vi "AddConnectionHandler.vi"(8 "error in (no error)":errorcluster, 11 "TCP_Server in":refnum<class "TCP_Server.lvclass">) -> (0 "error out":errorcluster, 3 "TCP_Server out":refnum<class "TCP_Server.lvclass">)   [LabVIEW 2023, in "TCP_Server.lvlib" / "TCP_Server.lvclass"]
uses:
  TCP_Server.lvclass
  TCP_Server_Connection_Handler/TCP_Server_Connection_Handler/TCP_Server_Connection_Handler.lvclass
  TCP_Server.lvclass/TCP_Server.ctl
  TCP_Server_Connection_Handler/TCP_Server_Connection_Handler Messages/Write Connection Information Msg/Write Connection Information Msg.lvclass/Write Connection Information Msg.ctl
  <vilib>/ActorFramework/Message Enqueuer/Message Enqueuer.lvclass/Message Enqueuer.ctl
  <vilib>/ActorFramework/Actor/Actor.lvclass/Actor.ctl
  TCP_Server_Connection_Handler/TCP_Server_Connection_Handler Messages/Write Error Logger's Enqueuer Msg/Write Error Logger's Enqueuer Msg.lvclass/Write Error Logger's Enqueuer Msg.ctl
  <vilib>/ActorFramework/Message Enqueuer/Enqueue.vi
  <vilib>/ActorFramework/Message Enqueuer/Init from Existing Queue.vi
  TCP_Server_Connection_Handler/TCP_Server_Connection_Handler Messages/Write Connection Information Msg/Write Connection Information Msg.lvclass
  TCP_Server_Connection_Handler/TCP_Server_Connection_Handler Messages/Write Error Logger's Enqueuer Msg/Write Error Logger's Enqueuer Msg.lvclass
  TCP_Server_Connection_Handler/TCP_Server_Connection_Handler Messages/FindMessageStart Msg/FindMessageStart Msg.lvclass
  TCP_Server Messages/AddConnectionWindow Msg/AddConnectionWindow Msg.lvclass
  <vilib>/ActorFramework/Message Priority Queue/Priority Enqueue.vi
  <vilib>/ActorFramework/Message Enqueuer/Message Enqueuer.lvclass
  <vilib>/ActorFramework/Actor/Actor.lvclass
  TCP_Server_Connection_Handler/TCP_Server_Connection_Handler Messages/SendWelcome Msg/SendWelcome Msg.lvclass
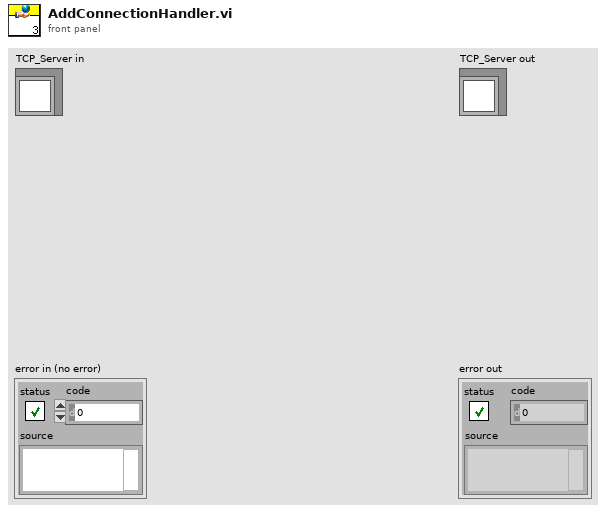
[diagram p1: front panel]
types:
  T1 = typedef "TCP_Server.lvlib/ServerConnection.ctl" = cluster{"Connection Handlers's Enqueuer":refnum<class "Message Enqueuer.lvclass">, "Connection Window's Enqueuer":refnum<class "Message Enqueuer.lvclass">, "Connection Information":T2}
  T2 = typedef "TCP_Listener.lvlib/ConnectionInformation.ctl" = cluster{"Connection number":i32, "Remote Address":string, "Remote Port":u16, "Connection ID":refnum<k5>}
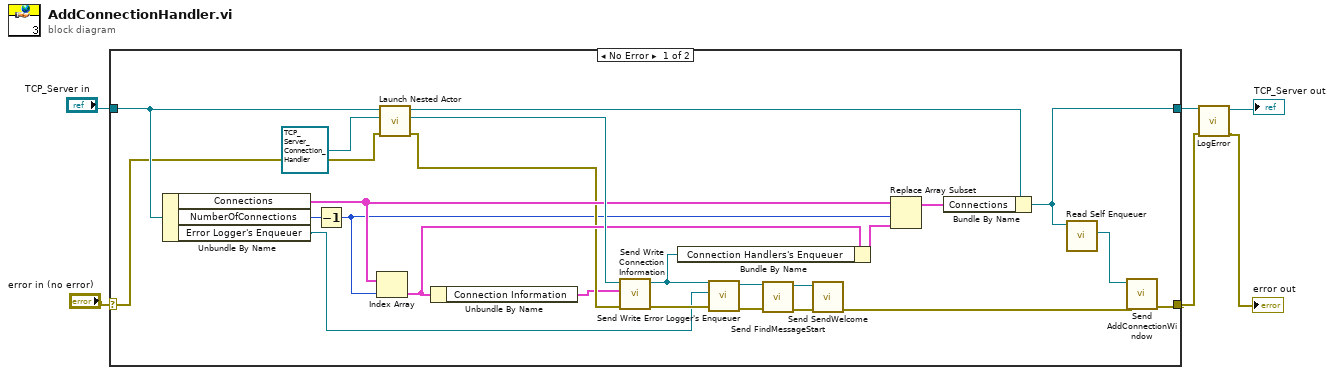
[diagram p0: block diagram]
diagram:
  n1 = case shown="No Error" "error in (no error)" {
    selector: "error in (no error)" -> [w18 w32]
    tunnel: [w20 w32] -> w2
    tunnel: [w19 w31] -> w4
    tunnel: "TCP_Server in" -> [w25 w31]
    frame No Error {
      n2 = Unbundle By Name(w25) -> ("Connections"=w23:T1[], "NumberOfConnections"=w29:i32, "Error Logger's Enqueuer"=w12:refnum<class "Message Enqueuer.lvclass">)
      n3 = Decrement(x=w29) -> (x-1=w15:i32)
      n4 = Index Array(array=w23, index=w15) -> (element=w21:T1)
      n5 = call <vilib>:"Launch Nested Actor.vi"("error in (no error)"=w18, "Nested Actor"=refnum<class "TCP_Server_Connection_Handler.lvclass"> refnum ("TCP_Server_Connection_Handler.lvlib:TCP_Server_Connection_Handler.lvclass"), "Caller Actor in"=w25) -> ("error out"=w17:errorcluster, "Nested Actor's Enqueuer"=w28:refnum<class "Message Enqueuer.lvclass">, "Caller Actor out"=w27:refnum<class "TCP_Server.lvclass">)  [unwired: 6 in]
      n6 = Unbundle By Name(w21) -> ("Connection Information"=w16:T2)
      n7 = call "Send Write Connection Information.vi"("error in (no error)"=w17, "Connection Information"=w16, "Message Enqueuer"=w28) -> ("error out"=w13:errorcluster, "Message Enqueuer out"=w14:refnum<class "Message Enqueuer.lvclass">)  [unwired: 7 in]
      n8 = Bundle By Name(cluster=w21, "Connection Handlers's Enqueuer"=w14) -> (w22:T1)
      n9 = call "Send Write Error Logger's Enqueuer.vi"("error in (no error)"=w13, "Actor Framework:Message Enqueuer"=w12, "Message Enqueuer"=w14) -> ("error out"=w11:errorcluster, "Message Enqueuer out"=w10:refnum<class "Message Enqueuer.lvclass">)  [unwired: 7 in]
      n10 = call "Send FindMessageStart.vi"("error in (no error)"=w11, "Message Enqueuer"=w10) -> ("error out"=w9:errorcluster, "Message Enqueuer out"=w8:refnum<class "Message Enqueuer.lvclass">)  [unwired: 8 in]
      n11 = call "Send SendWelcome.vi"("error in (no error)"=w9, "Message Enqueuer"=w8) -> ("error out"=w7:errorcluster)  [unwired: 8 in, 1 out]
      n12 = Replace Array Subset(array=w23, new element=w22, index=w15) -> (w26:T1[])
      n13 = Bundle By Name(cluster=w27, "Connections"=w26) -> (w19:refnum<class "TCP_Server.lvclass">)
      n14 = call <vilib>:"Read Self Enqueuer.vi"("Actor"=w19) -> ("Self Enqueuer"=w24:refnum<class "Message Enqueuer.lvclass">)  [unwired: 10 in]
      n15 = call "Send AddConnectionWindow.vi"("error in (no error)"=w7, "Message Enqueuer"=w24) -> ("error out"=w20:errorcluster)  [unwired: 8 in, 1 out]
    }
    frame Error {
    }
  }
  n16 = call "LogError.vi"("error in (no error)"=w2, "TCP_Server in"=w4) -> ("error out"=→"error out":errorcluster, "TCP_Server out"=→"TCP_Server out":refnum<class "TCP_Server.lvclass">)  [unwired: 8 in]
